vi "LoopselFFramp.VI"() -> ()   [LabVIEW 2015]
uses:
  <vilib>/Analysis/NI_AALBase.lvlib
panel:
  out "variance":dbl=1706837.362727273
  out "standard deviation":dbl=1306.459858827386
  out "mean":dbl=4072.47
  in  "Pixel":u16
  in  "DO8":u16
  in  "TO8":u16
  in  "D02":u16=100
  in  "Send O CTRL":bool
  in  "TM0H":u16
  in  "TM0L":u16=1000
  in  "DO7":u16
  in  "TO7":u16
  in  "DO6":u16
  in  "TO6":u16
  in  "DO5":u16
  in  "TO5":u16
  in  "DO4":u16
  in  "T04":u16
  in  "DO3":u16
  in  "TO3":u16
  in  "TO2":u16=10
  in  "Arm/Clear arry":bool
  in  "Start Read":bool
  in  "?":enum32{"1", "2", "3"}(radio)=enum."3"
  in  "pos slope":u8=1
  in  "both slopes":u8
  in  "DAT in 10ns":u32
  out "FIFO overflow":bool
  in  "extTrig 0/1":u8
  in  "Start Read":bool
  in  "stop all":bool
  in  "Arm/Clear arry":bool
  in  "Slide":u32(slide)=507 scale=1.0..1000.0
  in  "frequency[Hz]":u32
  in  "no.of samples (nos)":u32=1000
  in  "exposuretime[ms]":dbl=1.0 format="%.3f"
  out "Signalverlaufgraph":u16[](graph)=[3970, 3970, 3970, 3970, 0, 1, 0, 92, 6396, 6715, 6657, 6409, 7165, 6843, 7085, 6347, 6363, 6161, 6677, 6709, 6669, 6591, 7033, 6981, 7073, 6585, 6925, 7509, 6581, 7437, 7273, 6829, 6883, 7185, 6453, 6219, 7219, 6727, 6933, 6249, 7255, 6575, 6337, 6867, 6617, 6307, 7081, 7119, 6653, 6367, 7237, 7911, 6559, 6697, 6775, 7929, 6725, 7451, 6749, 6047, 7067, 6963, 6805, 7305, 6799, 6643, 6939, 6991, 6553, 7681, 6163, 6653, 6829, 7775, 6571, 6709, 6195, 6273, 7403, 6737, 7177, 6669, 7247, 6819, 6759, 6839, 6463, 6565, 7193, 6805, 6487, 6939, 6847, 6883, 6623, 7061, 6425, 6785, 6825, 7663, 7193, 6981, 6951, 6813, 6103, 6847, 7117, 6517, 6629, 7723, 6669, 6351, 6853, 6767, 6707, 6709, 6777, 6887, 6599, 6437, 6565, 6667, 6445, 6521, 6399, 6329, 6717, 7363, 7589, 7365, 6575, 7127, 6211, 6335, 6383, 4845, 4845, 5768, 6237, 6209, 5901, 5909, 6699, 5921, 5841, 5837, 5881, 6083, 6805, 6447, 6123, 6695, 6403, 5661, 6647, 6071, 6561, 6027, 6163, 6125, 5749, 7029, 6189, 6081, 6461, 6861, 5809, 6055, 6517, 6301, 6603, 6173, 6535, 6311, 6775, 6185, 7149, 7109, 5819, 6241, 6379, 6135, 6151, 6357, 6201, 6101, 6241, 6589, 6817, 6471, 6923, 6199, 6211, 6231, 6501, 6307, 6545, 7095, 6193, 6871, 6121, 7031, 6735, 5489, 6513, 6321, 5761, 6413, 6295, 6201, 6643, 6737, 6503, 6169, 6599, 5769, 6161, 6383, 6345, 6571, 6571, 6175, 6091, 6191, 5973, 5715, 5859, 6181, 6775, 6151, 6121, 5817, 6387, 6005, 6765, 6407, 6087, 6189, 6175, 6515, 6867, 6169, 6113, 6441, 6599, 6745, 6009, 6285, 6163, 5853, 6071, 6269, 5789, 5463, 6471, 6631, 6369, 6029, 6317, 5677, 6621, 5993, 6061, 6057, 6057, 5660, 5839, 5617, 5775, 5697, 5301, 5997, 5351, 6549, 5693, 5847, 5791, 5637, 5471, 5541, 5673, 5939, 5797, 5927, 6445, 5945, 6239, 6097, 5783, 5653, 6445, 6063, 5973, 5637, 6339, 6027, 5531, 5721, 5693, 6095, 6347, 6085, 6365, 5799, 5461, 5729, 5729, 6299, 6025, 5683, 6071, 5623, 5685, 5719, 6085, 5491, 5719, 5917, 5189, 5879, 6769, 5497, 6257, 5687, 5537, 6295, 5645, 6389, 5957, 6617, 6023, 5951, 5939, 5983, 6573, 5499, 5797, 6095, 5989, 5681, 6131, 5891, 6173, 6427, 5889, 6239, 5339, 5797, 5755, 5507, 5993, 6281, 6709, 5705, 5751, 5995, 5975, 6033, 5987, 6613, 5539, 6415, 6093, 6169, 6463, 6125, 5769, 5623, 5871, 5759, 5771, 5919, 6281, 5475, 6155, 5817, 5683, 5675, 5477, 5899, 5935, 6441, 5759, 5811, 5673, 5889, 5769, 5359, 5539, 5809, 5497, 5303, 5303, 5416, 6085, 5831, 5719, 5675, 5719, 5625, 6113, 5821, 6485, 6467, 5915, 6833, 6145, 5839, 6247, 6009, 6319, 5979, 6355, 5703, 6833, 6037, 6121, 5947, 6325, 6441, 6063, 6701, 6179, 6077, 6649, 6589, 6601, 6005, 6037, 5691, 5749, 6647, 6271, 6349, 5429, 6617, 6163, 5775, 6437, 6145, 5927, 6149, 6315, 6029, 6041, 5607, 5739, 6369, 6415, 6221, 6895, 6105, 6207, 6067, 6221, 6579, 6611, 6133, 6063, 6355, 6321, 6653, 6013, 6583, 5863, 5979, 6037, 6525, 5585, 6663, 6231, 6175, 6163, 7223, 5369, 6113, 6261, 5693, 6229, 6631, 7021, 5995, 6329, 6619, 6543, 7569, 6345, 5719, 6145, 6819, 5663, 6551, 7119, 6617, 6203, 6705, 6945, 6083, 6319, 6471, 6249, 6473, 6435, 6599, 5799, 5753, 5935, 6437, 6299, 6455, 6823, 6269, 5745, 6239, 6263, 5897, 6119, 6075, 6355, 6043, 6043, 6092, 6917, 7223, 7623, 6571, 7851, 7683, 7627, 7791, 7411, 7389, 7039, 7301, 7731, 7333, 8497, 7085, 8631, 7731, 8003, 8151, 7325, 7295, 7793, 7691, 7847, 7655, 7585, 8403, 7771, 8507, 8539, 7883, 7431, 7975, 7897, 8621, 7423, 7463, 8483, 7521, 8425, 7687, 8463, 7199, 8291, 7243, 7703, 7433, 7881, 7101, 8903, 7795, 7483, 7973, 7351, 7237, 7667, 6725, 7467, 8229, 7589, 7735, 8051, 7431, 8299, 7585, 7587, 6891, 7305, 7463, 7909, 8095, 7729, 7717, 7761, 7935, 8013, 9061, 8539, 8003, 8901, 8507, 7833, 7995, 8113, 7693, 8083, 8047, 8221, 6991, 8613, 7927, 7643, 7351, 7481, 7829, 7723, 8223, 8581, 7029, 7895, 7495, 6513, 7323, 8047, 7079, 7729, 8389, 8263, 8659, 8257, 7115, 7725, 7623, 8171, 8173, 7421, 7257, 7935, 7861, 8221, 7983, 8249, 6863, 7575, 7643, 7643, 5676, 5879, 5843, 5253, 5665, 5749, 5451, 6219, 5671, 5763, 6409, 5451, 5987, 5605, 6659, 5857, 6395, 5677, 5661, 5723, 5955, 6659, 6285, 7031, 6195, 5821, 6231, 5917, 5927, 5207, 6053, 5877, 6399, 6345, 6911, 6007, 6621, 6163, 5605, 6237, 6005, 5949, 5973, 5917, 5799, 6251, 6417, 6735, 6633, 5813, 5879, 6455, 6133, 6145, 6375, 5643, 5911, 6659, 6113, 6505, 5849, 6013, 6115, 6325, 6555, 6249, 6453, 6485, 6787, 5899, 6651, 6471, 5725, 5941, 6175, 6399, 6027, 6455, 7183, 6657, 6067, 6037, 6419, 6427, 5891, 6295, 5983, 6535, 6335, 5729, 6963, 6661, 6487, 5675, 5977, 6057, 6193, 6657, 6887, 6931, 5751, 6419, 6337, 6819, 7137, 6141, 6891, 5873, 6181, 5749, 6029, 6281, 6131, 6551, 5861, 5731, 6091, 6485, 6681, 6017, 6321, 5589, 6965, 6405, 6085, 6797, 6963, 6963, 6008, 6307, 6455, 6689, 6437, 6285, 6921, 6917, 6805, 6227, 6287, 6341, 6725, 6339, 7331, 6823, 6629, 7333, 6491, 6673, 6599, 7137, 6773, 6975, 6785, 6925, 7131, 6779, 7467, 6691, 7929, 6905, 6367, 6795, 6543, 7049, 6239, 6705, 6657, 7033, 7161, 6689, 7509, 6437, 7349, 6673, 6855, 6493, 7129, 6851, 6829, 6649, 6433, 6931, 7273, 7989, 6513, 7507, 6261, 7473, 6885, 6695, 7441, 6773, 7155, 6995, 6389, 6433, 7461, 6685, 6955, 6707, 7301, 6595, 6991, 6533, 7091, 7827, 6971, 6863, 7067, 6969, 7439, 6133, 6513, 6315, 6591, 5975, 8043, 6607, 6837, 7003, 6901, 6403, 7195, 6297, 7955, 6553, 8651, 6485, 6819, 6953, 7237, 6975, 7253, 7559, 6759, 6767, 6351, 7129, 7949, 6707, 7717, 6803, 7117, 6797, 6999, 6591, 7155, 7967, 7043, 6507, 7457, 6911, 7077, 6347, 6815, 6815, 6550, 7753, 7605, 8217, 7911, 8267, 8043, 7227, 8087, 9275, 7877, 7701, 7371, 8355, 8349, 7657, 8661, 7829, 7839, 7703, 7255, 7349, 7565, 8055, 8247, 8061, 8581, 8233, 8161, 7801, 7213, 8793, 8541, 8925, 9029, 8155, 7575, 8179, 8989, 7707, 8289, 8823, 8571, 7873, 8259, 8959, 7369, 8117, 7447, 6871, 8475, 8613, 8751, 8483, 8191, 7897, 8201, 7579, 7987, 8731, 9197, 8203, 9199, 8195, 8419, 7833, 8397, 8435, 8467, 9167, 8475, 7633, 7097, 7781, 8393, 9205, 8305, 8761, 10093, 8933, 7951, 8219, 8305, 8467, 7575, 7519, 8711, 8825, 7203, 7789, 7505, 8817, 8395, 8325, 7703, 8297, 7235, 8103, 7743, 8807, 8751, 7881, 8739, 7823, 8627, 7945, 8653, 8175, 9535, 7057, 8639, 8291, 8619, 7729, 8019, 8423, 8497, 8601, 9301, 8461, 9109, 8299, 8093, 9097, 8965, 8975, 9583, 9583, 3968, 4022, 3948, 3958, 3958, 3958, 3958, 3958, 3958, 3958, 3958, 3958, 3958, 3958, 3958, 3958, 3958, 3958, 3958, 3958, 3958, 3958, 3958, 3958, 3958, 3958, 3958, 3958, 3958, 3958, 3958, 3958, 3958, 3958, 3958, 3958, 3958, 3958, 3958, 3958, 3958, 3958, 3958, 3958, 3958, 3958, 3958, 3958, 3958, 3958, 3958, 3958, 3958, 3958, 3958]
  # "Start with run"
  # "Tn: delay"
  # "Abort with ESC"
  # "Dn: duration"
  # "*5ns"
  # "TO1: T0 main clock"
  # "period"
  # "*10ns"
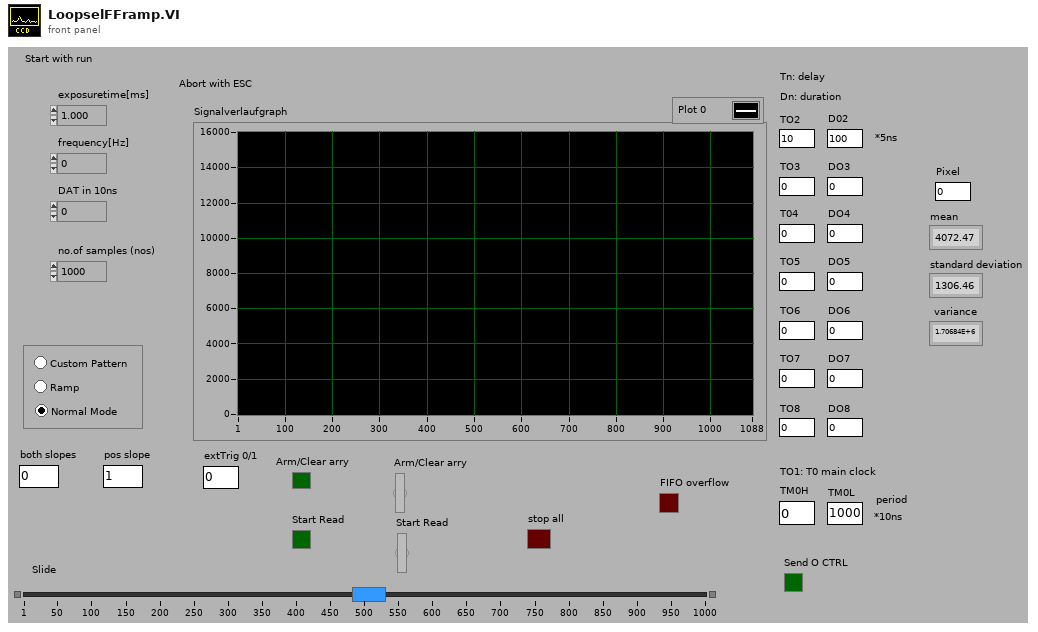
[diagram p1: front panel]
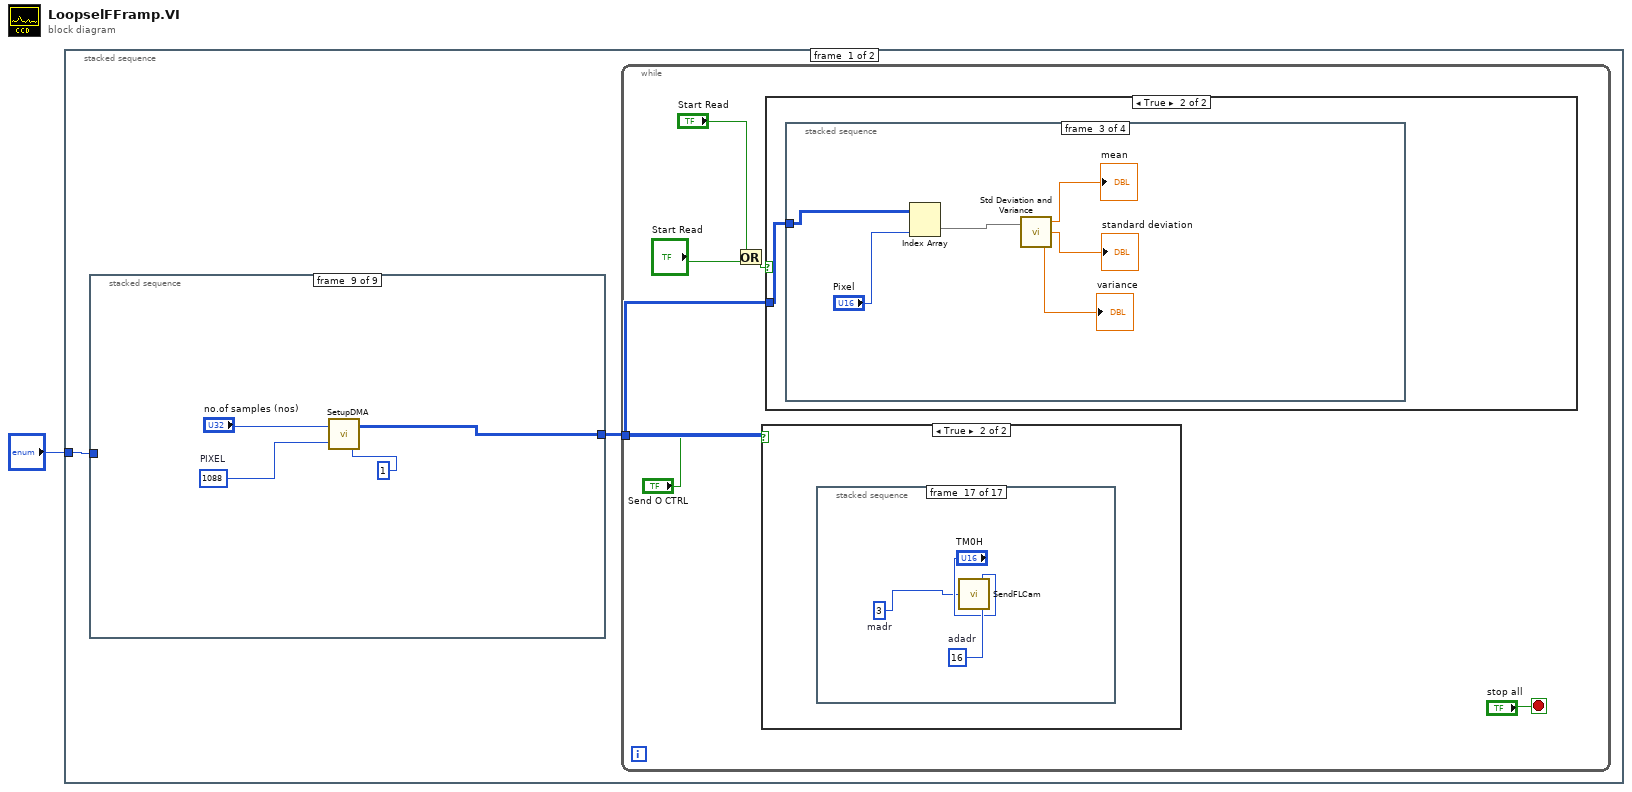
[diagram p0: block diagram]
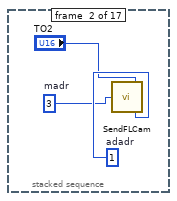
[diagram p4: hidden frame]
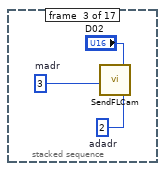
[diagram p5: hidden frame]
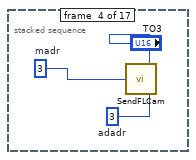
[diagram p6: hidden frame]
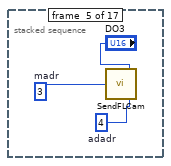
[diagram p7: hidden frame]
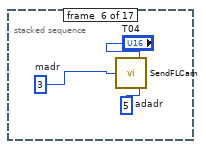
[diagram p8: hidden frame]
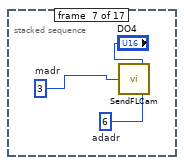
[diagram p9: hidden frame]
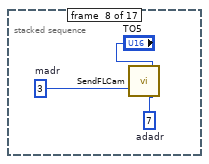
[diagram p10: hidden frame]
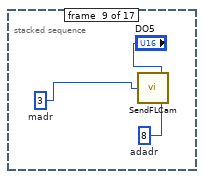
[diagram p11: hidden frame]
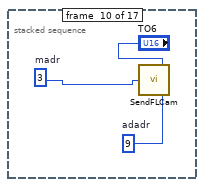
[diagram p12: hidden frame]
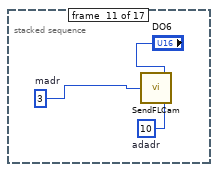
[diagram p13: hidden frame]
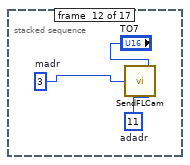
[diagram p14: hidden frame]
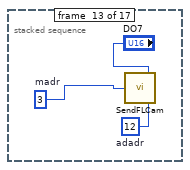
[diagram p15: hidden frame]
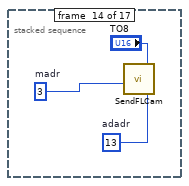
[diagram p16: hidden frame]
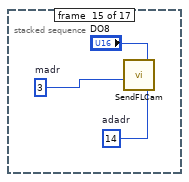
[diagram p17: hidden frame]
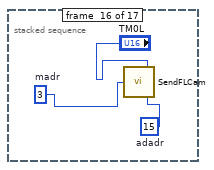
[diagram p18: hidden frame]
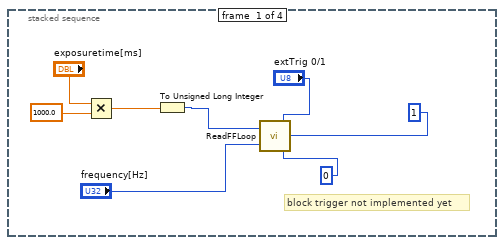
[diagram p20: hidden frame]
diagram:
  n1 = stacked-sequence {
    tunnel: "?" -> [w2 _]
    frame #0 {
      n2 = stacked-sequence {
        tunnel: [_ _ _ _ _ _ _ _ w125] -> w3
        tunnel: w2 -> [_ _ _ _ w91 _ _ _ _]
        frame #0 {
          n3 = call "InitDrv.vi"() -> ()  [unwired: 1 in]
        }
        frame #1 {
          # "pixel"
          # "xckdelay"
          # "A/D: 2=8bit, 1=12/16bit"
          n4 = call "InitBrd.vi"("xckdly"=u32 0, "pixel"=u32 1088, "flag816"=u32 1) -> ()  [unwired: 3 in]
        }
        frame #2 {
          n5 = case shown="1" "both slopes" {
            frame 0, Default {
              n6 = case shown="1" "pos slope" {
                frame 0, Default {
                  n7 = call "LowSlope.vi"() -> ()  [unwired: 1 in]
                }
                frame 1 {
                  n8 = call "HiSlope.vi"() -> ()  [unwired: 1 in]
                }
              }
            }
            frame 1 {
              n9 = call "BothSlopes.vi"() -> ()  [unwired: 1 in]
            }
          }
        }
        frame #3 {
          # "set TrigOut plug to show:"
          # "if (fkt==0)set to XCK -> XCK\nif (fkt==1)set to REG -> OutTrig\nif (fkt==2)set to FFRead\nif (fkt==3)set toTrigIn\nif (fkt==4)set to XCKDLY\nif (fkt==5)set to DAT"
          n10 = call "SetTOREG.vi"("fkt"=u8 0) -> ()
        }
        frame #4 {
          n11 = case shown="\"3\"" w91 {
            frame "1" {
              w92 = 0  # data
              w93 = 38  # adadr
              w94 = 1  # madr
              w95 = 18  # data
              w96 = 37  # adadr
              w97 = 1  # madr
              # "Custom Pattern"
              n12 = call "SendFLCam.vi"("madr"=w97, "data"=w95, "adadr"=w96) -> ()
              n13 = call "SendFLCam.vi"("madr"=w94, "data"=w92, "adadr"=w93) -> ()
            }
            frame "2" {
              w98 = 64  # data
              w99 = 37  # adadr
              w100 = 1  # madr
              # "Ramp"
              n14 = call "SendFLCam.vi"("madr"=w100, "data"=w98, "adadr"=w99) -> ()
            }
            frame "3" {
              w101 = 1  # data
              w103 = 0  # adadr
              w102 = 1  # madr
              w106 = 0  # data
              w105 = 38  # adadr
              w104 = 1  # madr
              w109 = 0  # data
              w108 = 37  # adadr
              w107 = 1  # madr
              # "Normal Mode"
              n15 = call "SendFLCam.vi"("madr"=w104, "data"=w106, "adadr"=w105) -> ()
              n16 = call "SendFLCam.vi"("madr"=w102, "data"=w101, "adadr"=w103) -> ()
              n17 = call "SendFLCam.vi"("madr"=w107, "data"=w109, "adadr"=w108) -> ()
            }
          }
        }
        frame #5 {
          w112 = 5000  # data
          w111 = 1  # adadr
          w110 = 3  # madr
          n18 = call "SendFLCam.vi"("madr"=w110, "data"=w112, "adadr"=w111) -> ()
        }
        frame #6 {
          # "bit31 must be set for enabling DAT(add 0x80000000) to REG 0x20"
          # "is only valid for external trigger!"
          # "this examples shows how to set the DAT (delay after trigger)"
          n19 = Equal To 0?(x="DAT in 10ns") -> (x = 0?=w114:bool)
          n20 = case shown="False" w114 {
            tunnel: "DAT in 10ns" -> [w115 _]
            frame False {
              n21 = Add(x=u32 2147483648, y=w115) -> (x+y=w118:u32)
              n22 = call "WriteL.vi"("val"=w118, "offset"=u32 32) -> ()
            }
            frame True {
              n23 = call "WriteL.vi"("val"=0, "offset"=u32 32) -> ()
            }
          }
        }
        frame #7 {
          # "set gain must be last in init sequence"
          n24 = call "SetAdGain.vi"("gain"=u8 2) -> ()  [unwired: 1 in]
        }
        frame #8 {
          w124 = u32 1088  # PIXEL
          n25 = call "SetupDMA.vi"("blocks"=1, "pixel"=w124, "nos"="no.of samples (nos)") -> ("Data Values"=w125:u16[][])
        }
      }
      n26 = while {
        tunnel: w3 -> [w9]
        stop <- "stop all" stop-if-true
        n27 = Or(x="Start Read", y="Start Read") -> (x .or. y?=w7:bool)
        n28 = case shown="True" "Send O CTRL" {
          frame False {
          }
          frame True {
            n29 = stacked-sequence {
              frame #0 {
              }
              frame #1 {
                w12 = 1  # adadr
                w11 = 3  # madr
                n30 = call "SendFLCam.vi"("madr"=w11, "data"="TO2", "adadr"=w12) -> ()
              }
              frame #2 {
                w14 = 2  # adadr
                w15 = 3  # madr
                n31 = call "SendFLCam.vi"("madr"=w15, "data"="D02", "adadr"=w14) -> ()
              }
              frame #3 {
                w18 = 3  # adadr
                w17 = 3  # madr
                n32 = call "SendFLCam.vi"("madr"=w17, "data"="TO3", "adadr"=w18) -> ()
              }
              frame #4 {
                w21 = 4  # adadr
                w20 = 3  # madr
                n33 = call "SendFLCam.vi"("madr"=w20, "data"="DO3", "adadr"=w21) -> ()
              }
              frame #5 {
                w24 = 5  # adadr
                w23 = 3  # madr
                n34 = call "SendFLCam.vi"("madr"=w23, "data"="T04", "adadr"=w24) -> ()
              }
              frame #6 {
                w27 = 6  # adadr
                w26 = 3  # madr
                n35 = call "SendFLCam.vi"("madr"=w26, "data"="DO4", "adadr"=w27) -> ()
              }
              frame #7 {
                w30 = 7  # adadr
                w29 = 3  # madr
                n36 = call "SendFLCam.vi"("madr"=w29, "data"="TO5", "adadr"=w30) -> ()
              }
              frame #8 {
                w33 = 8  # adadr
                w32 = 3  # madr
                n37 = call "SendFLCam.vi"("madr"=w32, "data"="DO5", "adadr"=w33) -> ()
              }
              frame #9 {
                w34 = 9  # adadr
                w36 = 3  # madr
                n38 = call "SendFLCam.vi"("madr"=w36, "data"="TO6", "adadr"=w34) -> ()
              }
              frame #10 {
                w39 = 10  # adadr
                w38 = 3  # madr
                n39 = call "SendFLCam.vi"("madr"=w38, "data"="DO6", "adadr"=w39) -> ()
              }
              frame #11 {
                w42 = 11  # adadr
                w41 = 3  # madr
                n40 = call "SendFLCam.vi"("madr"=w41, "data"="TO7", "adadr"=w42) -> ()
              }
              frame #12 {
                w45 = 12  # adadr
                w44 = 3  # madr
                n41 = call "SendFLCam.vi"("madr"=w44, "data"="DO7", "adadr"=w45) -> ()
              }
              frame #13 {
                w47 = 13  # adadr
                w48 = 3  # madr
                n42 = call "SendFLCam.vi"("madr"=w48, "data"="TO8", "adadr"=w47) -> ()
              }
              frame #14 {
                w50 = 14  # adadr
                w51 = 3  # madr
                n43 = call "SendFLCam.vi"("madr"=w51, "data"="DO8", "adadr"=w50) -> ()
              }
              frame #15 {
                w53 = 15  # adadr
                w54 = 3  # madr
                n44 = call "SendFLCam.vi"("madr"=w54, "data"="TM0L", "adadr"=w53) -> ()
              }
              frame #16 {
                w57 = 16  # adadr
                w55 = 3  # madr
                n45 = call "SendFLCam.vi"("madr"=w55, "data"="TM0H", "adadr"=w57) -> ()
              }
            }
          }
        }
        n46 = case shown="True" w7 {
          tunnel: w9 -> [_ w58]
          frame False {
          }
          frame True {
            n47 = stacked-sequence {
              tunnel: w58 -> [_ _ w75 w76]
              frame #0 {
                # "block trigger not implemented yet"
                n48 = Multiply(x="exposuretime[ms]", y=1000.0) -> (x*y=w66:dbl)
                n49 = To Unsigned Long Integer(number=w66) -> (unsigned 32bit integer=w63:u32)
                n50 = call "ReadFFLoop.vi"("exptus"=w63, "freq"="frequency[Hz]", "ExtTrig"="extTrig 0/1", "btrig_ch"=u32 1, "blocktrigger"=u8 0) -> ()
              }
              frame #1 {
                n51 = call "FFOvl.vi"() -> ("FFOvl"=w68:u8)  [unwired: 1 in]
                n52 = Not Equal?(x=w68, y=0) -> (x != y?=→"FIFO overflow":bool)
              }
              frame #2 {
                n53 = Index Array(array=w75, index (col)="Pixel") -> (element=w73:u16[])  [unwired: 1 in]
                n54 = call <vilib>:"Std Deviation and Variance.vi"("X"=w73) -> ("mean"=→"mean":dbl, "standard deviation"=→"standard deviation":dbl, "variance"=→"variance":dbl)  [unwired: 1 in]
              }
              frame #3 {
                n55 = while {
                  tunnel: w76 -> [w78]
                  stop <- w84 continue-if-true
                  n56 = Decrement(x="Slide") -> (x-1=w83:u32)
                  n57 = Index Array(array=w78, index (row)=w83) -> (element=→"Signalverlaufgraph":u16[])  [unwired: 1 in]
                  n58 = Or(x="Arm/Clear arry", y="Arm/Clear arry") -> (x .or. y?=w79:bool)
                  n59 = Not(x=w79) -> (.not. x?=w84:bool)
                }
              }
            }
          }
        }
      }
    }
    frame #1 {
      n60 = call "Exit.vi"() -> ()  [unwired: 1 in]
    }
  }
